vi "T1.vi"(9 "Sampling Frequency":dbl=100000000.0, 10 "Frequency":dbl, 11 "Line Code":string="11001101011") -> (2 "NumberOfSamplesPerBit":i32=26, 3 "Binary Waveform":dbl[](array[numeric]))   [LabVIEW 2018]
doc: "Generate T1 waveform."
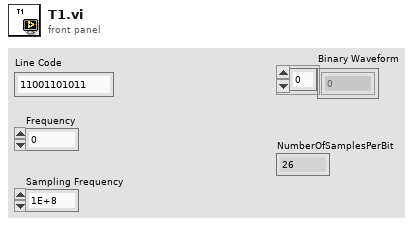
[diagram p1: front panel]
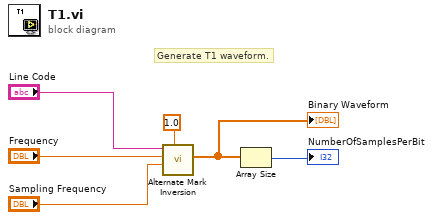
[diagram p0: block diagram]
diagram:
  # "Generate T1 waveform."
  n1 = call "Alternate Mark Inversion.vi"("Amplitude"=1.0, "Sampling Frequency"="Sampling Frequency", "Frequency"="Frequency", "Line Code"="Line Code") -> ("Signal"=w2:dbl[])  [unwired: 4 in, 3 out]
  "Binary Waveform" <- w2
  n2 = Array Size(array=w2) -> (size(s)=→"NumberOfSamplesPerBit":i32)
